vi "MGCC_EnergyMgmt_EMS_HTB.vi"() -> ()   [LabVIEW 2016]
uses:
  Communication/Global communication.vi
  Communication/Global communication output.vi
  <vilib>/imath/engines/lvmath2/RunTimeEngine/BuiltInFunctions/sum/NIMS_sum(GM,Sca).vi
  <instcachedir>/0/NIMS_sum(GM,Sca)_79BF37D5D11844228B167097B6AFCFEB.lvgen/NIMS_sum(GM,Sca)_79BF37D5D11844228B167097B6AFCFEB_001.vi
  <vilib>/imath/engines/lvmath2/RunTimeEngine/RangeToken/NIMS_Range_R2 - Integer.vi
  <instcachedir>/0/NIMS_Range_R2 - Integer_89B873E74E6E489885E44F751DD9C6BF.lvgen/NIMS_Range_R2 - Integer_89B873E74E6E489885E44F751DD9C6BF_000.vi
  <vilib>/imath/engines/lvmath2/RunTimeEngine/CommandStatement/MC_CommandStatement_break.vi
  <vilib>/imath/engines/lvmath2/RunTimeEngine/VariableToken/NIMS_VariableToken_CondDefinedDefinedByReplace.vi
  <instcachedir>/0/NIMS_VariableToken_CondDefinedDefinedByReplace_D162CFFC24174562A9FEA619A91E1A56.lvgen/NIMS_VariableToken_CondDefinedDefinedByReplace_D162CFFC24174562A9FEA619A91E1A56_003.vi
  <vilib>/imath/engines/lvmath2/RunTimeEngine/IndexRead/NIMS V(R2).vi
  <instcachedir>/0/NIMS V(R2)_C76619605A0E4E9F8B2FA9389712AC47.lvgen/NIMS V(R2)_C76619605A0E4E9F8B2FA9389712AC47_000.vi
  <vilib>/imath/engines/lvmath2/RunTimeEngine/BuiltInFunctions/sum/NIMS_sum(GV).vi
  <instcachedir>/0/NIMS_sum(GV)_67F5EC36BC034E54A6BEC5B0673C00E5.lvgen/NIMS_sum(GV)_67F5EC36BC034E54A6BEC5B0673C00E5_000.vi
  <vilib>/imath/engines/lvmath2/RunTimeEngine/IndexReplace/NIMS V(S)=S.vi
  <instcachedir>/0/NIMS V(S)=S_57E16554CB8B4B90AAB163894F717546.lvgen/NIMS V(S)=S_57E16554CB8B4B90AAB163894F717546_000.vi
  <vilib>/imath/engines/lvmath2/RunTimeEngine/ErrorHandling/NIMS_Create Error From Enums.vi
  <vilib>/imath/engines/lvmath2/RunTimeEngine/VariableToken/NIMS_VariableToken_CondDefined.vi
  <instcachedir>/0/NIMS_VariableToken_CondDefined_06E9DA95BD4D46A6BA55EC651A891960.lvgen/NIMS_VariableToken_CondDefined_06E9DA95BD4D46A6BA55EC651A891960_003.vi
  <vilib>/imathl/engines/lvmath/Functions/Error Handling/Create Error.vi
  <vilib>/imath/engines/lvmath2/RunTimeEngine/BuiltInFunctions/is_nan/NIMS_is_nan.vi
  <instcachedir>/0/NIMS_is_nan_BCCD798162CC49E3A8E57072444F6EB6.lvgen/NIMS_is_nan_BCCD798162CC49E3A8E57072444F6EB6_003.vi
  <vilib>/imath/engines/lvmath2/RunTimeEngine/BuiltInFunctions/max/1 input/NIMS_max(RV).vi
  <instcachedir>/0/NIMS_max(RV)_237633DB1D604D5BA7001287DF3C7957.lvgen/NIMS_max(RV)_237633DB1D604D5BA7001287DF3C7957_002.vi
  <vilib>/imath/engines/lvmath2/RunTimeEngine/BuiltInFunctions/tril/NIMS_tril.vi
  <instcachedir>/0/NIMS_tril_6D22CCA5CB604C1FB8874D0E0A590B2C.lvgen/NIMS_tril_6D22CCA5CB604C1FB8874D0E0A590B2C_003.vi
  <vilib>/imath/engines/lvmath2/RunTimeEngine/RowToken/NIMS_RowToken_M_CV.vi
  <instcachedir>/0/NIMS_RowToken_M_CV_FA79F1D1D17D44459F3ED8E09EE8B625.lvgen/NIMS_RowToken_M_CV_FA79F1D1D17D44459F3ED8E09EE8B625_002.vi
  <vilib>/imath/engines/lvmath2/RunTimeEngine/MatrixToken/NIMS_MatrixToken_M_M.vi
  <instcachedir>/0/NIMS_MatrixToken_M_M_DF273B0CC20F424BBF1EDA9F4E71C841.lvgen/NIMS_MatrixToken_M_M_DF273B0CC20F424BBF1EDA9F4E71C841_005.vi
  <vilib>/imath/engines/lvmath2/RunTimeEngine/ArithmeticOperatorToken/NIMS_ArithmeticOperator_minus.vi
  <instcachedir>/0/NIMS_ArithmeticOperator_minus_E3B65B1D26A44BB184AFDC5B3F458E3D.lvgen/NIMS_ArithmeticOperator_minus_E3B65B1D26A44BB184AFDC5B3F458E3D_003.vi
  <vilib>/imath/engines/lvmath2/RunTimeEngine/BuiltInFunctions/double/NIMS_double.vi
  <instcachedir>/0/NIMS_double_34E32F64C2B04A25A042F4CA881A0A41.lvgen/NIMS_double_34E32F64C2B04A25A042F4CA881A0A41_000.vi
  <instcachedir>/0/NIMS_double_34E32F64C2B04A25A042F4CA881A0A41.lvgen/NIMS_double_34E32F64C2B04A25A042F4CA881A0A41_002.vi
  <instcachedir>/0/NIMS_double_34E32F64C2B04A25A042F4CA881A0A41.lvgen/NIMS_double_34E32F64C2B04A25A042F4CA881A0A41_003.vi
  <vilib>/imath/engines/lvmath2/RunTimeEngine/RowToken/NIMS_RowToken_M_M.vi
  <instcachedir>/0/NIMS_RowToken_M_M_968CDE3545E74ACDAEA4B48DE01EEECA.lvgen/NIMS_RowToken_M_M_968CDE3545E74ACDAEA4B48DE01EEECA_004.vi
  <vilib>/imath/engines/lvmath2/RunTimeEngine/MatrixToken/NIMS_MatrixToken_M_RV.vi
  <instcachedir>/0/NIMS_MatrixToken_M_RV_EE14907D4B194E829889005D2F556E9C.lvgen/NIMS_MatrixToken_M_RV_EE14907D4B194E829889005D2F556E9C_001.vi
  <instcachedir>/0/NIMS_MatrixToken_M_M_DF273B0CC20F424BBF1EDA9F4E71C841.lvgen/NIMS_MatrixToken_M_M_DF273B0CC20F424BBF1EDA9F4E71C841_004.vi
  <vilib>/imath/engines/lvmath/Functions/Error Handling/MergeErrorsWrapper.vi
  <vilib>/imath/engines/lvmath2/RunTimeEngine/BuiltInFunctions/fmin_lp/NIMS_fmin_lp.vi
  <vilib>/imath/engines/lvmath2/RunTimeEngine/IndexRead/NIMS V(S).vi
  <instcachedir>/0/NIMS V(S)_0488751826AF41519A22953C041130DC.lvgen/NIMS V(S)_0488751826AF41519A22953C041130DC_000.vi
  <instcachedir>/0/NIMS_max(RV)_237633DB1D604D5BA7001287DF3C7957.lvgen/NIMS_max(RV)_237633DB1D604D5BA7001287DF3C7957_000.vi
  <vilib>/imath/engines/lvmath2/RunTimeEngine/NodeEndStatement/NIMS_NodeEndStatement_Output.vi
  <instcachedir>/0/NIMS_NodeEndStatement_Output_53EC0D466D134D7ABD903AC30B43404B.lvgen/NIMS_NodeEndStatement_Output_53EC0D466D134D7ABD903AC30B43404B_005.vi
  <instcachedir>/0/NIMS_NodeEndStatement_Output_53EC0D466D134D7ABD903AC30B43404B.lvgen/NIMS_NodeEndStatement_Output_53EC0D466D134D7ABD903AC30B43404B_001.vi
  <instcachedir>/0/NIMS_NodeEndStatement_Output_53EC0D466D134D7ABD903AC30B43404B.lvgen/NIMS_NodeEndStatement_Output_53EC0D466D134D7ABD903AC30B43404B_010.vi
  <vilib>/imath/engines/lvmath2/RunTimeEngine/ErrorHandling/NIMS_Finalize Error.vi
  CostSavings.vi
  Battery Dispatch.vi
  Load Forecasting (Mike)/Sub-VIs/CriticalLoadIndex.vi
  <instcachedir>/0/NIMS_RowToken_M_M_968CDE3545E74ACDAEA4B48DE01EEECA.lvgen/NIMS_RowToken_M_M_968CDE3545E74ACDAEA4B48DE01EEECA_005.vi
  <vilib>/imath/engines/lvmath2/RunTimeEngine/MatrixToken/NIMS_MatrixToken_M_SorCV.vi
  <instcachedir>/0/NIMS_MatrixToken_M_SorCV_D3266533510A4291A747E91CF193467A.lvgen/NIMS_MatrixToken_M_SorCV_D3266533510A4291A747E91CF193467A_001.vi
  <vilib>/imath/engines/lvmath2/RunTimeEngine/BuiltInFunctions/length/NIMS_length(GV).vi
  <instcachedir>/0/NIMS_length(GV)_08A3D13377FD4E4B96F5795FBF3698FA.lvgen/NIMS_length(GV)_08A3D13377FD4E4B96F5795FBF3698FA_002.vi
  <vilib>/imath/engines/lvmath2/RunTimeEngine/BuiltInFunctions/eye/NIMS_M=eye(I32).vi
  <instcachedir>/0/NIMS_NodeEndStatement_Output_53EC0D466D134D7ABD903AC30B43404B.lvgen/NIMS_NodeEndStatement_Output_53EC0D466D134D7ABD903AC30B43404B_002.vi
  Load Forecasting (Mike)/Sub-VIs/LoadCombinations.vi
  Load Forecasting (Mike)/Sub-VIs/SW_Combinations.vi
  <instcachedir>/0/NIMS_VariableToken_CondDefinedDefinedByReplace_D162CFFC24174562A9FEA619A91E1A56.lvgen/NIMS_VariableToken_CondDefinedDefinedByReplace_D162CFFC24174562A9FEA619A91E1A56_001.vi
  <vilib>/imath/engines/lvmath2/RunTimeEngine/IndexRead/NIMS M($,R2).vi
  <instcachedir>/0/NIMS M($,R2)_D9380E19261A4ADFB2D364AF6959C6EF.lvgen/NIMS M($,R2)_D9380E19261A4ADFB2D364AF6959C6EF_001.vi
  <vilib>/imath/engines/lvmath2/RunTimeEngine/IndexReplace/NIMS M($,S)=V.vi
  <instcachedir>/0/NIMS M($,S)=V_EEA74323A7E5479BB387BE0F93352290.lvgen/NIMS M($,S)=V_EEA74323A7E5479BB387BE0F93352290_001.vi
  <vilib>/imath/engines/lvmath2/RunTimeEngine/BuiltInFunctions/size/NIMS_[I32,I32]=size(GM).vi
  <instcachedir>/0/NIMS_[I32,I32]=size(GM)_B0A6EC1255BB4C8AB801FE6F734128D9.lvgen/NIMS_[I32,I32]=size(GM)_B0A6EC1255BB4C8AB801FE6F734128D9_005.vi
  <vilib>/imath/engines/lvmath2/RunTimeEngine/BuiltInFunctions/zeros/NIMS_M=zeros(I32,I32).vi
  <instcachedir>/0/NIMS_VariableToken_CondDefined_06E9DA95BD4D46A6BA55EC651A891960.lvgen/NIMS_VariableToken_CondDefined_06E9DA95BD4D46A6BA55EC651A891960_001.vi
  <vilib>/imath/engines/lvmath2/RunTimeEngine/IndexRead/NIMS M($,S).vi
  <instcachedir>/0/NIMS M($,S)_3E5749BBB62E49528D4765A77F1F6D98.lvgen/NIMS M($,S)_3E5749BBB62E49528D4765A77F1F6D98_000.vi
  <vilib>/imath/engines/lvmath2/RunTimeEngine/ArithmeticOperatorToken/NIMS_ArithmeticOperator_multmx(M,CV).vi
  <instcachedir>/0/NIMS_ArithmeticOperator_multmx(M,CV)_EE734FC8520844C9A7CC1A67008668A3.lvgen/NIMS_ArithmeticOperator_multmx(M,CV)_EE734FC8520844C9A7CC1A67008668A3_001.vi
  <vilib>/imath/engines/lvmath2/RunTimeEngine/BuiltInFunctions/ones/NIMS_V=ones(I32,I32).vi
  <instcachedir>/0/NIMS_ArithmeticOperator_minus_E3B65B1D26A44BB184AFDC5B3F458E3D.lvgen/NIMS_ArithmeticOperator_minus_E3B65B1D26A44BB184AFDC5B3F458E3D_002.vi
  <vilib>/imath/engines/lvmath2/RunTimeEngine/BuiltInFunctions/length/NIMS_length(GM).vi
  <instcachedir>/0/NIMS_length(GM)_47CEC356FCE0482D9BA47DC61C99F2C7.lvgen/NIMS_length(GM)_47CEC356FCE0482D9BA47DC61C99F2C7_000.vi
  <vilib>/imath/engines/lvmath2/RunTimeEngine/IndexRead/NIMS M(S).vi
  <instcachedir>/0/NIMS M(S)_B826C018497E4940AE96BD27B540B6FB.lvgen/NIMS M(S)_B826C018497E4940AE96BD27B540B6FB_000.vi
  <vilib>/imath/engines/lvmath2/RunTimeEngine/IndexReplace/NIMS M(S)=S.vi
  <instcachedir>/0/NIMS M(S)=S_B3274CDAFA9346529812A4A947D623CC.lvgen/NIMS M(S)=S_B3274CDAFA9346529812A4A947D623CC_001.vi
  <vilib>/imath/engines/lvmath2/RunTimeEngine/BuiltInFunctions/min/1 input/NIMS_min(RM).vi
  <instcachedir>/0/NIMS_min(RM)_55BCC15A0E9E4B598EACC10A12C4B58C.lvgen/NIMS_min(RM)_55BCC15A0E9E4B598EACC10A12C4B58C_000.vi
  <vilib>/imath/engines/lvmath2/RunTimeEngine/BuiltInFunctions/abs/NIMS_abs(signed).vi
  <instcachedir>/0/NIMS_abs(signed)_C4FCB8E6058B49B797C7C8D53CA5F6EC.lvgen/NIMS_abs(signed)_C4FCB8E6058B49B797C7C8D53CA5F6EC_005.vi
  <vilib>/imath/engines/lvmath2/RunTimeEngine/RelationalOperatorToken/NIMS_Relational_Operator_Eq.vi
  <instcachedir>/0/NIMS_Relational_Operator_Eq_FD198F059617437A8A02361002FCA645.lvgen/NIMS_Relational_Operator_Eq_FD198F059617437A8A02361002FCA645_004.vi
  <vilib>/imath/engines/lvmath2/RunTimeEngine/BuiltInFunctions/findnz/NIMS_[1o]_findnz(GM).vi
  <instcachedir>/0/NIMS_[1o]_findnz(GM)_0B85F0C1FD7A4D70A7D15487030BA0C8.lvgen/NIMS_[1o]_findnz(GM)_0B85F0C1FD7A4D70A7D15487030BA0C8_003.vi
  <vilib>/imath/engines/lvmath2/RunTimeEngine/BuiltInFunctions/is_empty/NIMS_is_empty(GM).vi
  <instcachedir>/0/NIMS_is_empty(GM)_AF8F13F4B7FD436CB1855477E2504B8A.lvgen/NIMS_is_empty(GM)_AF8F13F4B7FD436CB1855477E2504B8A_006.vi
  <instcachedir>/0/NIMS_VariableToken_CondDefinedDefinedByReplace_D162CFFC24174562A9FEA619A91E1A56.lvgen/NIMS_VariableToken_CondDefinedDefinedByReplace_D162CFFC24174562A9FEA619A91E1A56_004.vi
  <vilib>/imath/engines/lvmath2/RunTimeEngine/IndexRead/NIMS M(M,$).vi
  <instcachedir>/0/NIMS M(M,$)_85DD0EB51D694ED1820EB297DFD8A1B6.lvgen/NIMS M(M,$)_85DD0EB51D694ED1820EB297DFD8A1B6_004.vi
  <vilib>/imath/engines/lvmath2/RunTimeEngine/IndexReplace/NIMS M(S,$)=M.vi
  <instcachedir>/0/NIMS M(S,$)=M_47BFD2E070824516B94BE47F5466D205.lvgen/NIMS M(S,$)=M_47BFD2E070824516B94BE47F5466D205_000.vi
  <vilib>/imath/engines/lvmath2/RunTimeEngine/IndexReplace/NIMS V(S)=M.vi
  <instcachedir>/0/NIMS V(S)=M_6FB28FD48A0B4397A1C8FAEC68D14DDE.lvgen/NIMS V(S)=M_6FB28FD48A0B4397A1C8FAEC68D14DDE_001.vi
  <instcachedir>/0/NIMS_VariableToken_CondDefined_06E9DA95BD4D46A6BA55EC651A891960.lvgen/NIMS_VariableToken_CondDefined_06E9DA95BD4D46A6BA55EC651A891960_009.vi
  <instcachedir>/0/NIMS_NodeEndStatement_Output_53EC0D466D134D7ABD903AC30B43404B.lvgen/NIMS_NodeEndStatement_Output_53EC0D466D134D7ABD903AC30B43404B_015.vi
  <instcachedir>/0/NIMS_MatrixToken_M_SorCV_D3266533510A4291A747E91CF193467A.lvgen/NIMS_MatrixToken_M_SorCV_D3266533510A4291A747E91CF193467A_002.vi
  <vilib>/imath/engines/lvmath2/RunTimeEngine/BuiltInFunctions/zeros/NIMS_V=zeros(I32,I32).vi
  <vilib>/Utility/error.llb/Error Cluster From Error Code.vi
  <vilib>/ErrorRing/Error Ring.xnode
panel:
  out "Dispatched loads":dbl[](graph)
  out "Dispatched PV ISD":dbl[](graph)
  out "Crit_Ind":i32[](array[numeric])
  out "Forecast PV":dbl[](graph)
  out "Forecast Load":dbl[](graph)
  out "Battery Dispatch":dbl[](graph)
  out "Net load after":dbl[](graph)
  out "Net load b4":dbl[](graph)
  out "Savings":dbl
  out "error out ISD":errorcluster
  out "ISD_EMS_BATT":dbl[](array[numeric])
  out "ISD_EMS_PV":dbl[](array[numeric])
  out "Load_Forecast_GC":dbl[][](array[numeric])
  out "P_batt":dbl[](array[numeric])
  out "PV_Forecast_GC":dbl[](array[numeric])
  out "error out GC":errorcluster
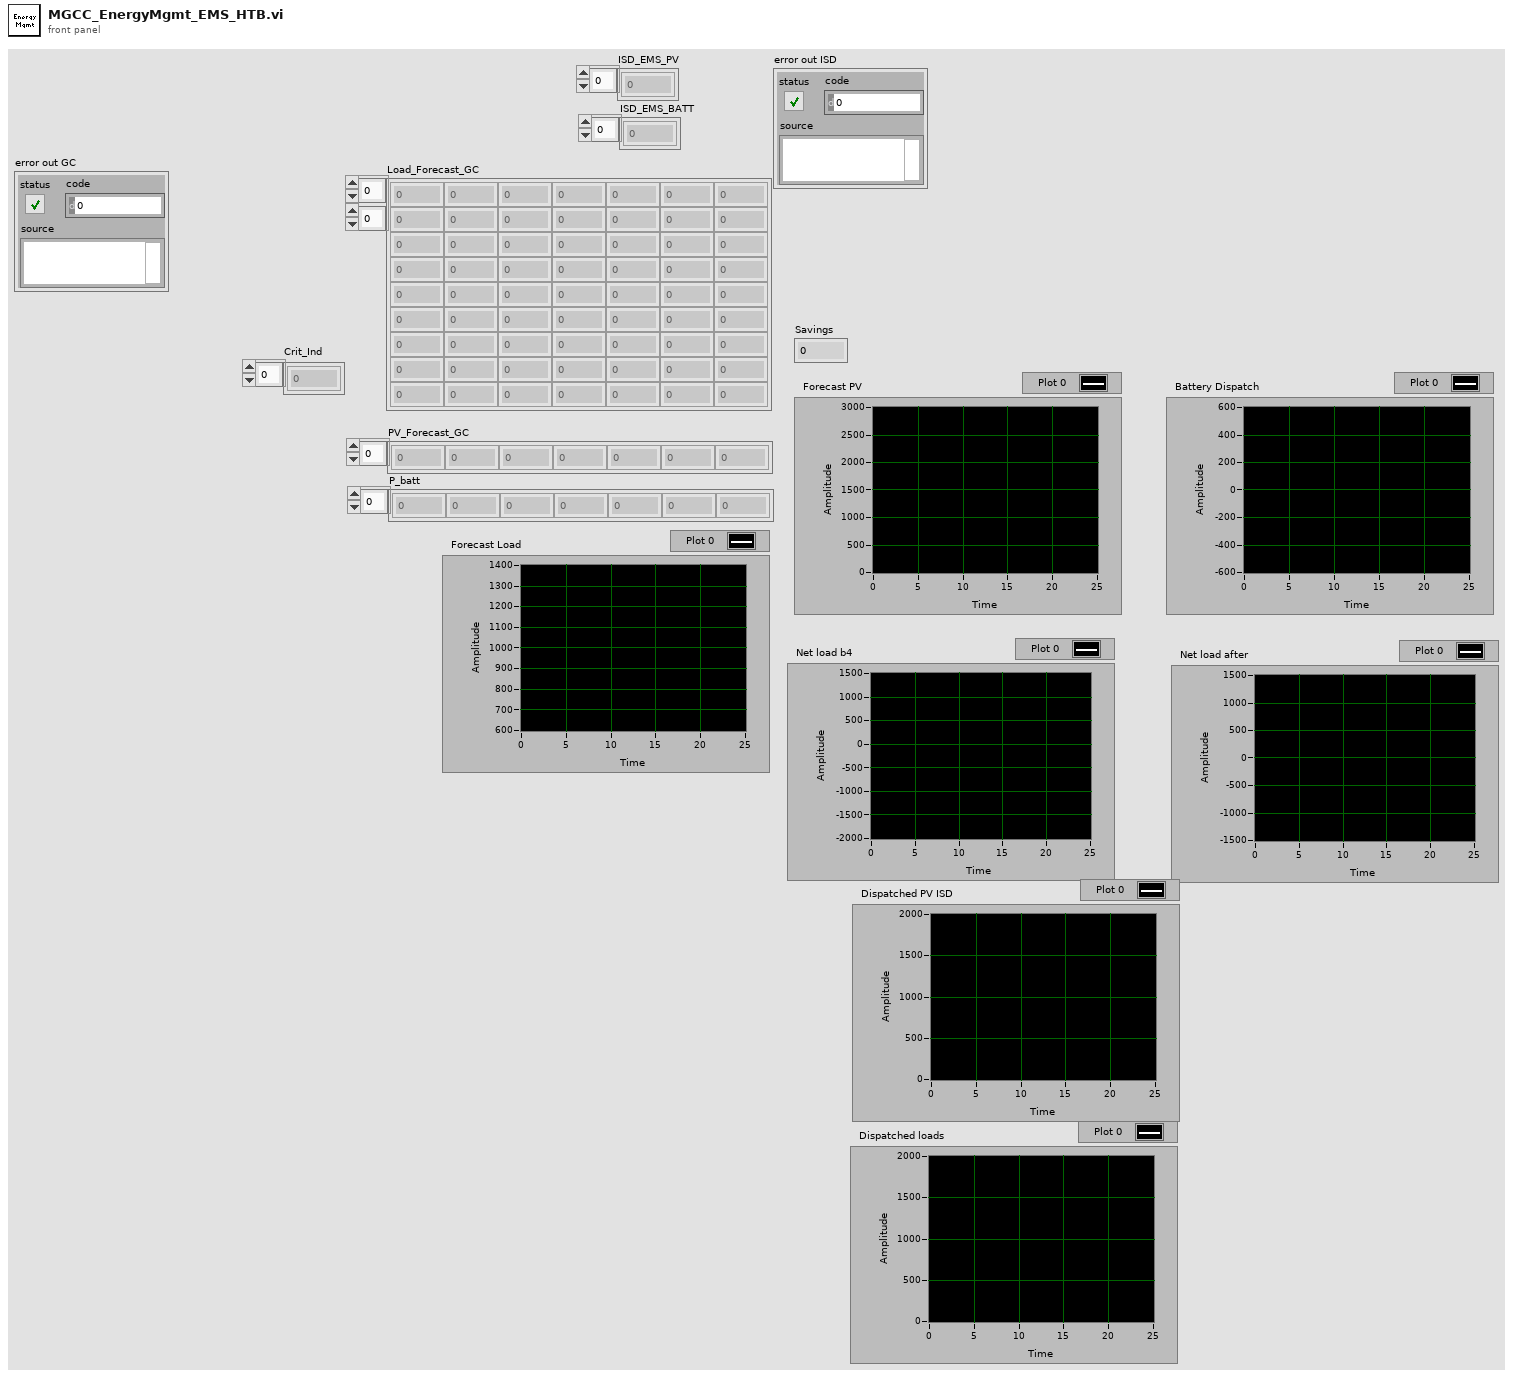
[diagram p1: front panel]
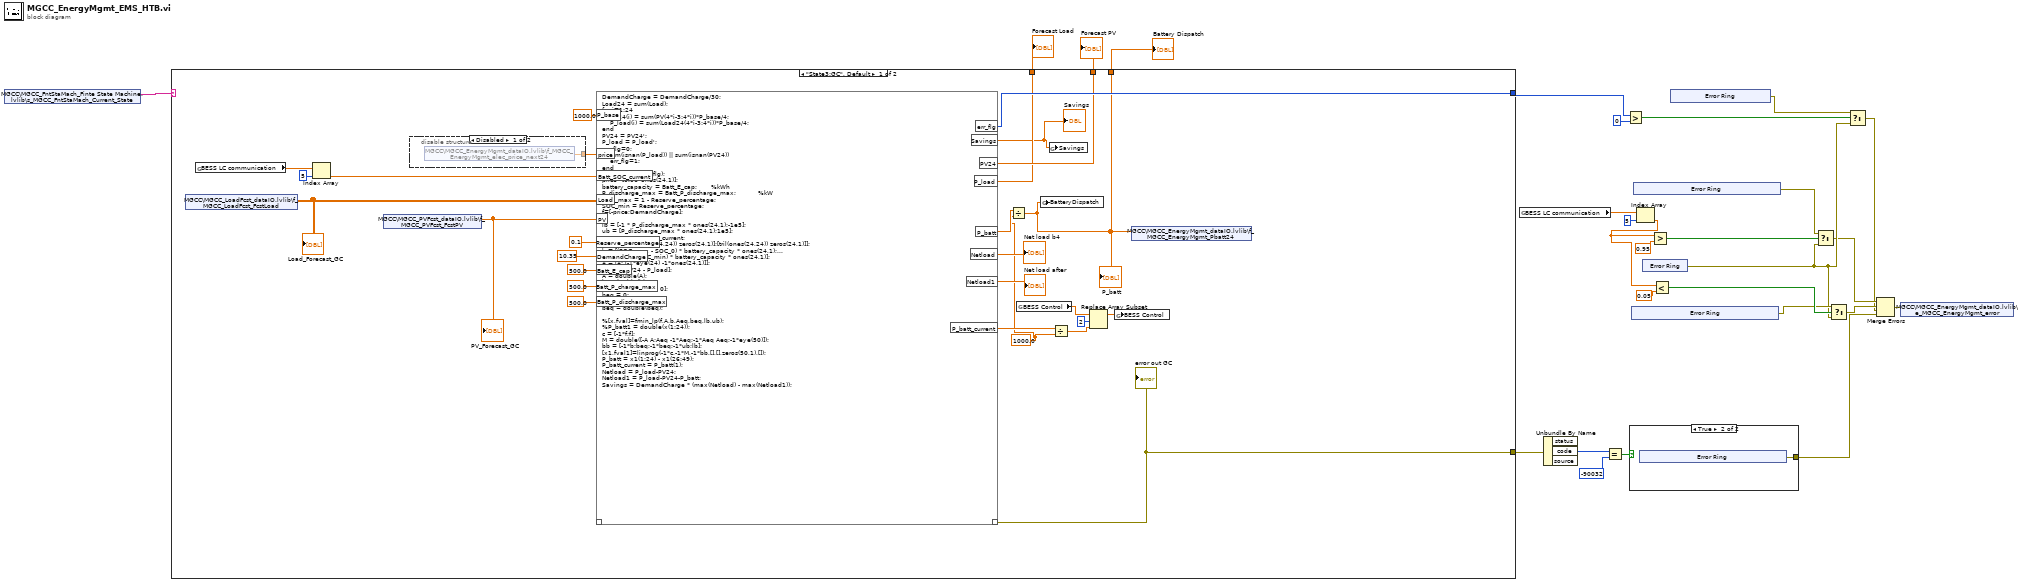
[diagram p0: block diagram]
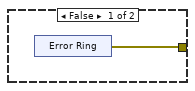
[diagram p2: hidden frame]
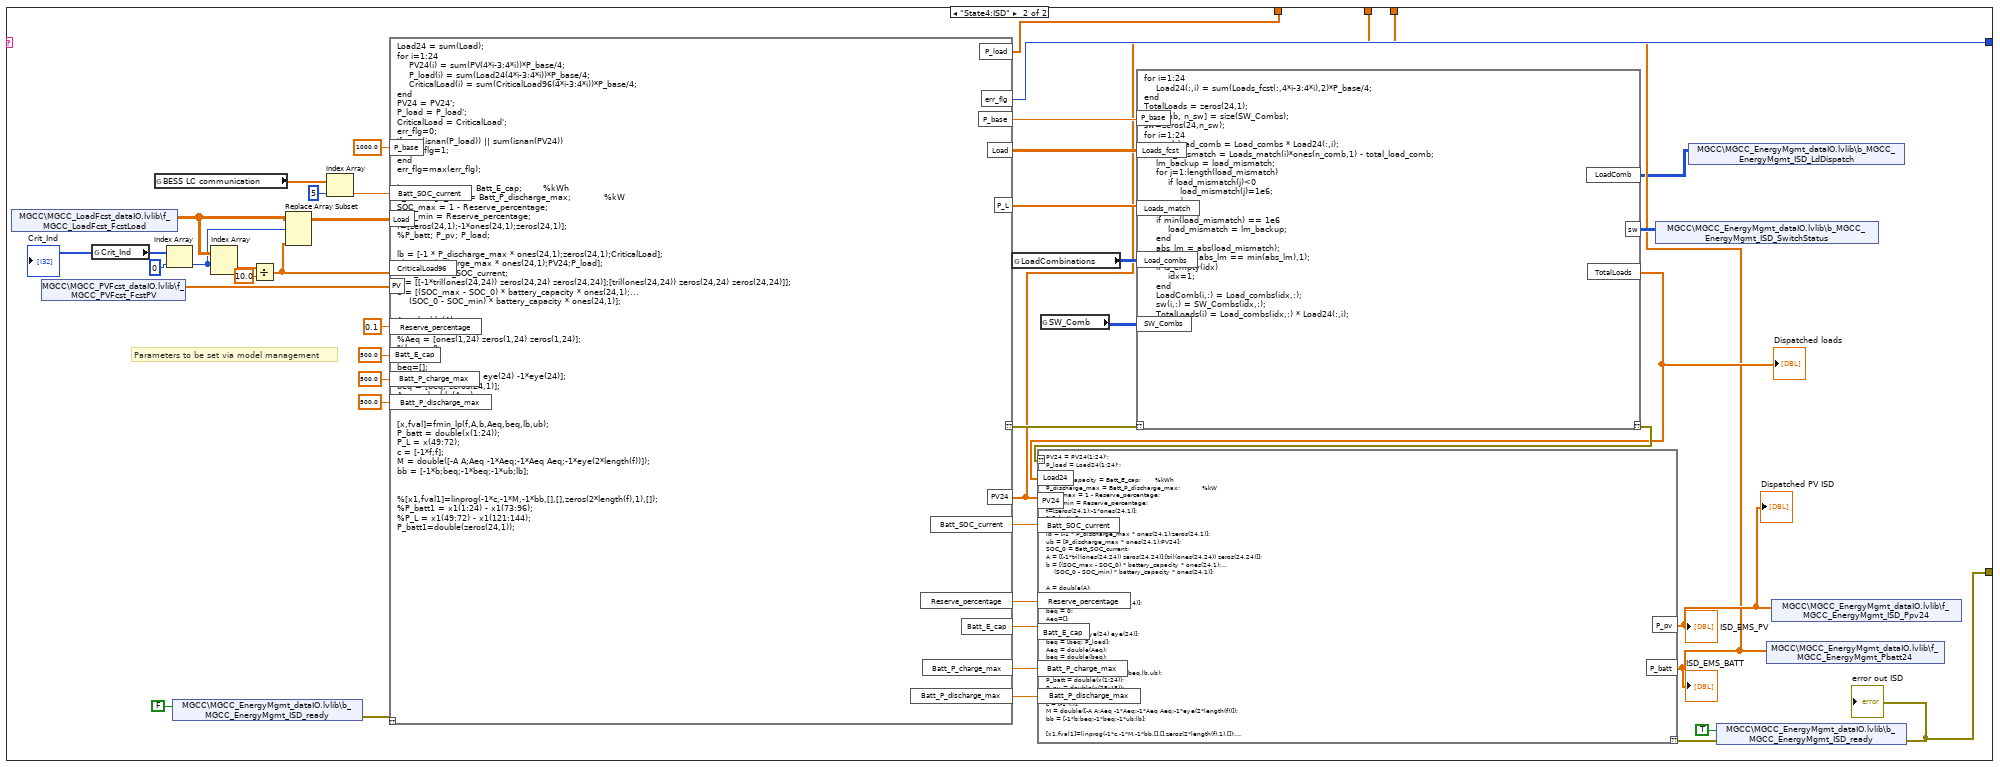
[diagram p4: hidden frame]
diagram:
  n1 = shared-variable "MGCC\\MGCC_FntStaMach_Finte State Machine.lvlib\\s_MGCC_FntStaMach_Current_State"() -> (w27:string)  [unwired: 1 in, 1 out]
  n2 = case shown="\"State3:GC\", Default" w27 {
    tunnel: [w46 w760] -> w19
    tunnel: [w36 w744] -> w5
    tunnel: [w33 w735] -> w8
    tunnel: [w32 w736] -> w7
    tunnel: [w28 w733] -> w6
    frame "State3:GC", Default {
      w29 = 1000.0 ("y")
      n3 = shared-variable "MGCC\\MGCC_LoadFcst_dataIO.lvlib\\f_MGCC_LoadFcst_FcstLoad"() -> (w45:dbl[][])  [unwired: 1 in, 1 out]
      "Load_Forecast_GC" <- w45
      n4 = global read "Global communication.vi" "BESS LC communication"() -> (w44:dbl[])
      n5 = Index Array(array=w44, index=5) -> (element=w42:dbl)
      n6 = shared-variable "MGCC\\MGCC_PVFcst_dataIO.lvlib\\f_MGCC_PVFcst_FcstPV"() -> (w49:dbl[])  [unwired: 1 in, 1 out]
      "PV_Forecast_GC" <- w49
      n7 = disable-structure shown="Disabled" {
        disable-tunnel: [w55 _] -> w54
        frame Disabled {
          n8 = shared-variable "MGCC\\MGCC_EnergyMgmt_dataIO.lvlib\\f_MGCC_EnergyMgmt_elec_price_next24"() -> (w55:dbl[])  [unwired: 1 in, 1 out]
        }
        frame Enabled {
        }
      }
      n9 = mathscript code="DemandCharge = DemandCharge/30;\nLoad24 = sum(Load);\nfor i=1:24\n    PV24(i) = sum(PV(4*i-3:4*i))*P_base/4;\n    P_load(i) = sum(Load24(4*i-3:4*i))*P_base/4;\nend\nPV24 = PV24';\nP_load = P_load';\nerr_flg=0;\nif sum(isnan(P_load)) || sum(isnan(PV24))\n    err_flg=1;\nend\nerr_flg=max(err_flg);\nprice=[0.06*ones(24,1)];\nbattery_capacity = Batt_E_cap;       %kWh\nP_discharge_max = Batt_P_discharge_max;           %kW\nSOC_max = 1 - Reserve_percentage;\nSOC_min = Reserve_percentage;\nf=[-price;DemandCharge];\n\nlb = [-1 * P_discharge_max * ones(24,1);-1e5];\nub = [P_discharge_max * ones(24,1);1e5];\nSOC_0 = Batt_SOC_current;\nA = [[-1*tril(ones(24,24)) zeros(24,1)];[tril(ones(24,24)) zeros(24,1)]];\nb = [(SOC_max - SOC_0) * battery_capacity * ones(24,1);...\n    (SOC_0 - SOC_min) * battery_capacity * ones(24,1)];\nA = [A; [-1*eye(24) -1*ones(24,1)]];\nb = [b; PV24 - P_load];\nA = double(A);\nb = double(b);\nAeq = [ones(1,24) 0];\nbeq = 0;\nAeq = double(Aeq);\nbeq = double(beq);\n\n%[x,fval]=fmin_lp(f,A,b,Aeq,beq,lb,ub);\n%P_batt1 = double(x(1:24));\nc = [-1*f;f];\nM = double([-A A;Aeq -1*Aeq;-1*Aeq Aeq;-1*eye(50)]);\nbb = [-1*b;beq;-1*beq;-1*ub;lb];\n[x1,fval1]=linprog(-1*c,-1*M,-1*bb,[],[],zeros(50,1),[]);\nP_batt = x1(1:24) - x1(26:49);\nP_batt_current = P_batt(1);\nNetload = P_load-PV24;\nNetload1 = P_load-PV24-P_batt;\nSavings = DemandCharge * (max(Netload) - max(Netload1));"("price"=w54, "Batt_E_cap"=500.0, "Batt_P_charge_max"=500.0, "Batt_P_discharge_max"=500.0, "Batt_SOC_current"=w42, "DemandCharge"=10.35, "Load"=w45, "PV"=w49, "Reserve_percentage"=0.1, "P_base"=1000.0) -> ("??"=w36:errorcluster, "P_batt"=w30:dbl[], "P_batt_current"=w47:dbl, "err_flg"=w46:i32, "Savings"=w31:dbl, "PV24"=w33:dbl[], "P_load"=w32:dbl[], "Netload"=→"Net load b4":dbl[], "Netload1"=→"Net load after":dbl[])  [unwired: 1 in]
      "error out GC" <- w36
      "Savings" <- w31
      n10 = Divide(x=w30, y=w29) -> (x/y=w28:dbl[])
      "P_batt" <- w28
      n11 = global read "Global communication output.vi" "BESS Control"() -> (w41:dbl[])
      n12 = global write "Battery Dispatch.vi" "BatteryDispatch"(w28) -> ()
      n13 = global write "CostSavings.vi" "Savings"(w31) -> ()
      n14 = Divide(x=w47, y=w29) -> (x/y=w39:dbl)
      n15 = Replace Array Subset(array=w41, new element=w39, index=2) -> (w38:dbl[])
      n16 = global write "Global communication output.vi" "BESS Control"(w38) -> ()
      n17 = shared-variable "MGCC\\MGCC_EnergyMgmt_dataIO.lvlib\\f_MGCC_EnergyMgmt_Pbatt24"(w28) -> ()  [unwired: 1 in, 1 out]
    }
    frame "State4:ISD" {
      # "Parameters to be set via model management"
      n18 = shared-variable "MGCC\\MGCC_LoadFcst_dataIO.lvlib\\f_MGCC_LoadFcst_FcstLoad"() -> (w743:dbl[][])  [unwired: 1 in, 1 out]
      n19 = shared-variable "MGCC\\MGCC_PVFcst_dataIO.lvlib\\f_MGCC_PVFcst_FcstPV"() -> (w767:dbl[])  [unwired: 1 in, 1 out]
      n20 = global read "CriticalLoadIndex.vi" "Crit_Ind"() -> (w766:i32[])
      "Crit_Ind" <- w766
      n21 = global read "Global communication.vi" "BESS LC communication"() -> (w772:dbl[])
      n22 = Index Array(array=w766, index=0) -> (element=w742:i32)
      n23 = shared-variable "MGCC\\MGCC_EnergyMgmt_dataIO.lvlib\\b_MGCC_EnergyMgmt_ISD_ready"(FALSE ("b_MGCC_EnergyMgmt_ISD_ready")) -> (error out=w768:errorcluster)  [unwired: 1 in]
      n24 = Index Array(array=w743, index (row)=w742) -> (element=w741:dbl[])  [unwired: 1 in]
      n25 = Divide(x=w741, y=10.0) -> (x/y=w739:dbl[])
      n26 = Replace Array Subset(array=w743, new element=w739, index (row)=w742) -> (w738:dbl[][])  [unwired: 1 in]
      n27 = Index Array(array=w772, index=5) -> (element=w770:dbl)
      n28 = mathscript code="Load24 = sum(Load);\nfor i=1:24\n    PV24(i) = sum(PV(4*i-3:4*i))*P_base/4;\n    P_load(i) = sum(Load24(4*i-3:4*i))*P_base/4;\n    CriticalLoad(i) = sum(CriticalLoad96(4*i-3:4*i))*P_base/4;\nend\nPV24 = PV24';\nP_load = P_load';\nCriticalLoad = CriticalLoad';\nerr_flg=0;\nif sum(isnan(P_load)) || sum(isnan(PV24))\n    err_flg=1;\nend\nerr_flg=max(err_flg);\n\nbattery_capacity = Batt_E_cap;       %kWh\nP_discharge_max = Batt_P_discharge_max;           %kW\nSOC_max = 1 - Reserve_percentage;\nSOC_min = Reserve_percentage;\nf=[zeros(24,1);-1*ones(24,1);zeros(24,1)];\n%P_batt; P_pv; P_load;\n\nlb = [-1 * P_discharge_max * ones(24,1);zeros(24,1);CriticalLoad];\nub = [P_discharge_max * ones(24,1);PV24;P_load];\nSOC_0 = Batt_SOC_current;\nA = [[-1*tril(ones(24,24)) zeros(24,24) zeros(24,24)];[tril(ones(24,24)) zeros(24,24) zeros(24,24)]];\nb = [(SOC_max - SOC_0) * battery_capacity * ones(24,1);...\n    (SOC_0 - SOC_min) * battery_capacity * ones(24,1)];\n\nA = double(A);\nb = double(b);\n%Aeq = [ones(1,24) zeros(1,24) zeros(1,24)];\n%beq = 0;\nAeq=[];\nbeq=[];\nAeq = [Aeq; eye(24) eye(24) -1*eye(24)];\nbeq = [beq; zeros(24,1)];\nAeq = double(Aeq);\nbeq = double(beq);\n\n[x,fval]=fmin_lp(f,A,b,Aeq,beq,lb,ub);\nP_batt = double(x(1:24));\nP_L = x(49:72);\nc = [-1*f;f];\nM = double([-A A;Aeq -1*Aeq;-1*Aeq Aeq;-1*eye(2*length(f))]);\nbb = [-1*b;beq;-1*beq;-1*ub;lb];\n\n\n%[x1,fval1]=linprog(-1*c,-1*M,-1*bb,[],[],zeros(2*length(f),1),[]);\n%P_batt1 = x1(1:24) - x1(73:96);\n%P_L = x1(49:72) - x1(121:144);\nP_batt1=double(zeros(24,1));"("??"=w768, "Batt_E_cap"=500.0, "Batt_P_charge_max"=500.0, "Batt_P_discharge_max"=500.0, "Batt_SOC_current"=w770, "Load"=w738, "PV"=w767, "Reserve_percentage"=0.1, "CriticalLoad96"=w739, "P_base"=1000.0) -> ("??"=w753:errorcluster, "P_L"=w759:dbl[], "err_flg"=w760:i32, "Load"=w756:dbl[][], "P_base"=w755:dbl, "PV24"=w735:dbl[], "Batt_SOC_current"=w751:dbl, "Reserve_percentage"=w750:dbl, "Batt_E_cap"=w749:dbl, "Batt_P_charge_max"=w748:dbl, "Batt_P_discharge_max"=w747:dbl, "P_load"=w736:dbl[])
      n29 = global read "LoadCombinations.vi" "LoadCombinations"() -> (w758:i32[][])
      n30 = global read "SW_Combinations.vi" "SW_Comb"() -> (w757:i32[][])
      n31 = mathscript code="for i=1:24\n    Load24(:,i) = sum(Loads_fcst(:,4*i-3:4*i),2)*P_base/4;\nend\nTotalLoads = zeros(24,1);\n[n_comb, n_sw] = size(SW_Combs);\nsw=zeros(24,n_sw);\nfor i=1:24\n    total_load_comb = Load_combs * Load24(:,i);\n    load_mismatch = Loads_match(i)*ones(n_comb,1) - total_load_comb;\n    lm_backup = load_mismatch;\n    for j=1:length(load_mismatch)\n        if load_mismatch(j)<0\n            load_mismatch(j)=1e6;\n        end\n    end\n    if min(load_mismatch) == 1e6\n        load_mismatch = lm_backup;\n    end\n    abs_lm = abs(load_mismatch);\n    idx = find(abs_lm == min(abs_lm),1);\n    if is_empty(idx)\n        idx=1;\n    end\n    LoadComb(i,:) = Load_combs(idx,:);\n    sw(i,:) = SW_Combs(idx,:);\n    TotalLoads(i) = Load_combs(idx,:) * Load24(:,i);\nend"("??"=w753, "Loads_fcst"=w756, "Loads_match"=w759, "Load_combs"=w758, "SW_Combs"=w757, "P_base"=w755) -> ("??"=w752:errorcluster, "sw"=w754:i32[][], "TotalLoads"=w737:dbl[], "LoadComb"=w732:i32[][])
      "Dispatched loads" <- w737
      n32 = mathscript code="PV24 = PV24(1:24)';\nP_load = Load24(1:24)';\n\nbattery_capacity = Batt_E_cap;       %kWh\nP_discharge_max = Batt_P_discharge_max;           %kW\nSOC_max = 1 - Reserve_percentage;\nSOC_min = Reserve_percentage;\nf=[zeros(24,1);-1*ones(24,1)];\n%P_batt; P_pv; \n\nlb = [-1 * P_discharge_max * ones(24,1);zeros(24,1)];\nub = [P_discharge_max * ones(24,1);PV24];\nSOC_0 = Batt_SOC_current;\nA = [[-1*tril(ones(24,24)) zeros(24,24)];[tril(ones(24,24)) zeros(24,24)]];\nb = [(SOC_max - SOC_0) * battery_capacity * ones(24,1);...\n    (SOC_0 - SOC_min) * battery_capacity * ones(24,1)];\n\nA = double(A);\nb = double(b);\nAeq = [ones(1,24) zeros(1,24)];\nbeq = 0;\nAeq=[];\nbeq=[];\nAeq = [Aeq; eye(24) eye(24)];\nbeq = [beq; P_load];\nAeq = double(Aeq);\nbeq = double(beq);\n\n[x,fval]=fmin_lp(f,A,b,Aeq,beq,lb,ub);\nP_batt = double(x(1:24));\nP_pv = double(x(25:48));\n\nc = [-1*f;f];\nM = double([-A A;Aeq -1*Aeq;-1*Aeq Aeq;-1*eye(2*length(f))]);\nbb = [-1*b;beq;-1*beq;-1*ub;lb];\n\n[x1,fval1]=linprog(-1*c,-1*M,-1*bb,[],[],zeros(2*length(f),1),[]);\nP_batt1 = x1(1:24) - x1(49:72);\nP_pv1 = x1(25:48) - x1(73:96);\nP_batt1=double(zeros(24,1));\nP_pv1=double(zeros(24,1));"("??"=w752, "Batt_E_cap"=w749, "Batt_P_charge_max"=w748, "Batt_P_discharge_max"=w747, "Batt_SOC_current"=w751, "Load24"=w737, "PV24"=w735, "Reserve_percentage"=w750) -> ("??"=w745:errorcluster, "P_pv"=w734:dbl[], "P_batt"=w733:dbl[])
      "ISD_EMS_PV" <- w734
      "ISD_EMS_BATT" <- w733
      "Dispatched PV ISD" <- w734
      n33 = shared-variable "MGCC\\MGCC_EnergyMgmt_dataIO.lvlib\\b_MGCC_EnergyMgmt_ISD_SwitchStatus"(w754) -> ()  [unwired: 1 in, 1 out]
      n34 = shared-variable "MGCC\\MGCC_EnergyMgmt_dataIO.lvlib\\b_MGCC_EnergyMgmt_ISD_LdDispatch"(w732) -> ()  [unwired: 1 in, 1 out]
      n35 = shared-variable "MGCC\\MGCC_EnergyMgmt_dataIO.lvlib\\b_MGCC_EnergyMgmt_ISD_ready"(TRUE ("b_MGCC_EnergyMgmt_ISD_ready"), error in=w745) -> (error out=w744:errorcluster)
      "error out ISD" <- w744
      n36 = shared-variable "MGCC\\MGCC_EnergyMgmt_dataIO.lvlib\\f_MGCC_EnergyMgmt_Pbatt24"(w733) -> ()  [unwired: 1 in, 1 out]
      n37 = shared-variable "MGCC\\MGCC_EnergyMgmt_dataIO.lvlib\\f_MGCC_EnergyMgmt_ISD_Ppv24"(w734) -> ()  [unwired: 1 in, 1 out]
    }
  }
  "Forecast Load" <- w7
  "Forecast PV" <- w8
  "Battery Dispatch" <- w6
  n38 = global read "Global communication.vi" "BESS LC communication"() -> (w11:dbl[])
  n39 = Unbundle By Name(w5) -> ("code"=w4:i32)  [unwired: 2 out]
  n40 = Equal?(x=w4, y=-90032) -> (x = y?=w2:bool)
  n41 = Greater?(x=w19, y=0) -> (0:w18:bool)
  n42 = case shown="True" w2 {
    tunnel: [w2520 w2522] -> w1
    frame False {
      n43 = xnode "Error Ring"() -> ("error out"=w2520:errorcluster)
    }
    frame True {
      n44 = xnode "Error Ring"() -> ("error out"=w2522:errorcluster)
    }
  }
  n45 = xnode "Error Ring"() -> ("error out"=w21:errorcluster)
  n46 = xnode "Error Ring"() -> ("error out"=w23:errorcluster)
  n47 = Index Array(array=w11, index=5) -> (element=w9:dbl)
  n48 = xnode "Error Ring"() -> ("error out"=w16:errorcluster)
  n49 = Greater?(x=w9, y=0.95) -> (0:w24:bool)
  n50 = Less?(x=w9, y=0.05) -> (x < y?=w22:bool)
  n51 = xnode "Error Ring"() -> ("error out"=w17:errorcluster)
  n52 = Select(t=w23, s=w24, f=w16) -> (s? t:f=w15:errorcluster)
  n53 = Select(t=w21, s=w22, f=w16) -> (s? t:f=w14:errorcluster)
  n54 = Select(t=w17, s=w18, f=w16) -> (s? t:f=w13:errorcluster)
  n55 = Merge Errors(w15, w14, w13, w1) -> (w12:errorcluster)
  n56 = shared-variable "MGCC\\MGCC_EnergyMgmt_dataIO.lvlib\\e_MGCC_EnergyMgmt_error"(w12) -> ()  [unwired: 1 in, 1 out]
